vi "MotorInterface.vi"() -> ()   [LabVIEW 2021]
panel:
  out "Waveform Chart":dynamicdata(graph)
  out "Fault":bool
  out "Square":dynamicdata(graph)
  in  "Run Motor":bool
  in  "Frequency of Steps":dbl
  out "Direction Test\nPort 0_2":bool[](array[boolean])
  out "Reset Test\nPort 0_1":bool[](array[boolean])
  out "Enable Test\nPort 0_0":bool[](array[boolean])
  in  "Direction":bool caption="Direction\n(down is up)"
  in  "Reset":bool
  in  "Enable":bool
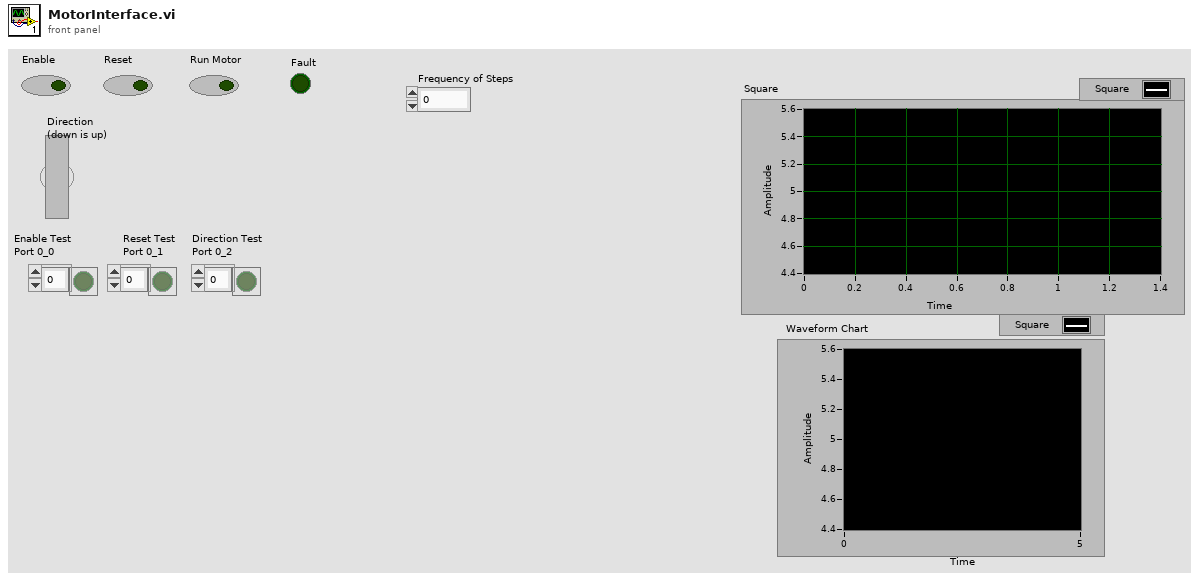
[diagram p1: front panel]
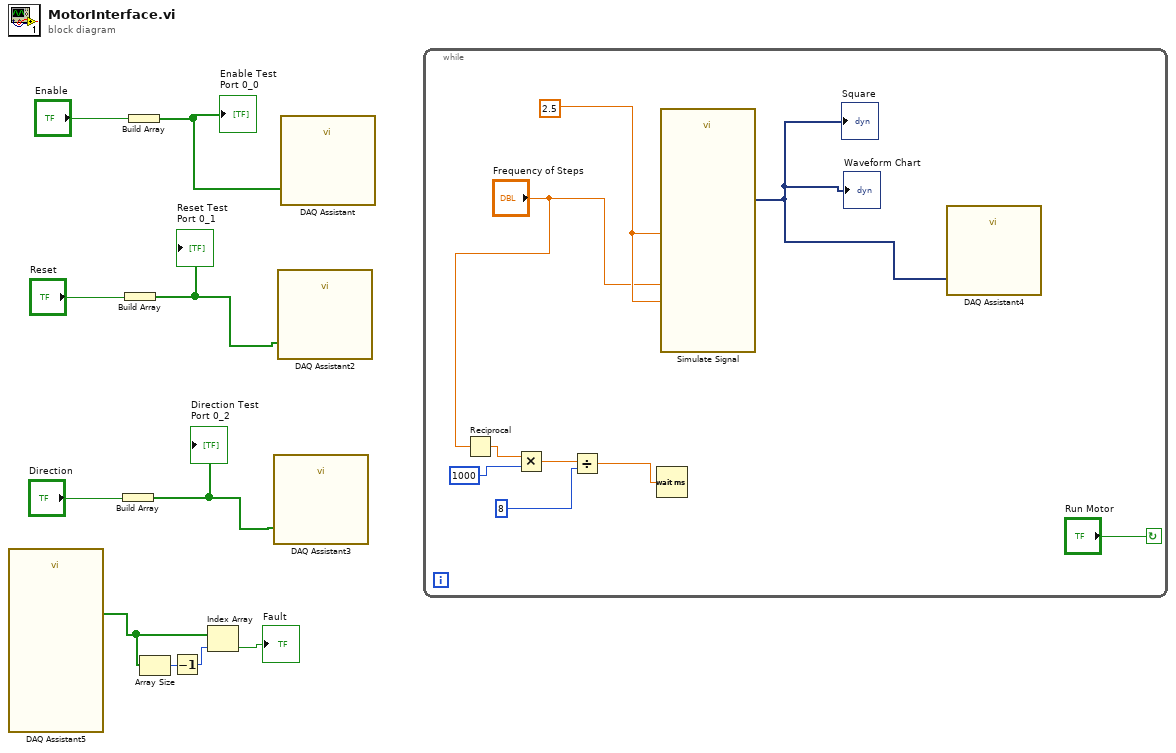
[diagram p0: block diagram]
diagram:
  n1 = call "DAQ Assistant5"() -> ("data"=w3:bool[])  [unwired: 17 in, 2 out]
  n2 = Build Array("Direction") -> (w5:bool[])
  "Direction Test\nPort 0_2" <- w5
  n3 = Build Array("Reset") -> (w7:bool[])
  "Reset Test\nPort 0_1" <- w7
  n4 = Build Array("Enable") -> (w10:bool[])
  "Enable Test\nPort 0_0" <- w10
  n5 = Array Size(array=w3) -> (size(s)=w2:i32)
  n6 = Decrement(x=w2) -> (x-1=w1:i32)
  n7 = Index Array(array=w3, index=w1) -> (element=→"Fault":bool)
  n8 = call "DAQ Assistant3"("data"=w5) -> ()  [unwired: 17 in, 2 out]
  n9 = call "DAQ Assistant2"("data"=w7) -> ()  [unwired: 17 in, 2 out]
  n10 = call "DAQ Assistant"("data"=w10) -> ()  [unwired: 17 in, 2 out]
  n11 = while {
    stop <- "Run Motor" continue-if-true
    w18 = 2.5
    n12 = Reciprocal(x="Frequency of Steps") -> (1/x=w16:dbl)
    n13 = Multiply(x=w16, y=1000) -> (x*y=w13:dbl)
    n14 = Divide(x=w13, y=8) -> (x/y=w12:dbl)
    n15 = Wait (ms)(milliseconds to wait=w12) -> ()  [unwired: 1 out]
    n16 = call "Simulate Signal"("Offset"=w18, "Frequency"="Frequency of Steps", "Amplitude"=w18) -> ("Square"=w11:dynamicdata)  [unwired: 11 in, 1 out]
    "Square" <- w11
    "Waveform Chart" <- w11
    n17 = call "DAQ Assistant4"("data"=w11) -> ()  [unwired: 16 in, 3 out]
  }
